vi "Set_Power_Unit.vi"(0 ".NET Reference in":refnum<k24>, 1 "unit":i32(ring) items=["dBm", "mW"], 3 "error in (no error)":errorcluster) -> (7 "Reference out":refnum<k24>, 10 "error out":errorcluster)   [LabVIEW 2017]
uses:
  LV_IL_Sample/DLL/InstrumentDLL.dll
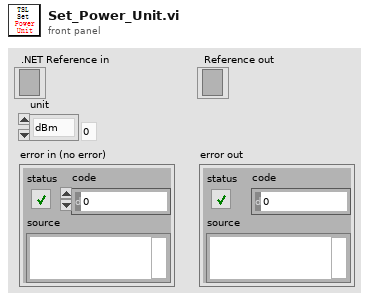
[diagram p1: front panel]
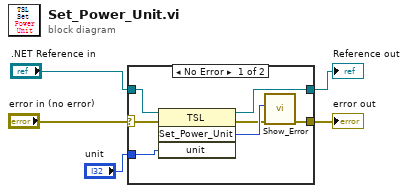
[diagram p0: block diagram]
diagram:
  n1 = case shown="No Error" "error in (no error)" {
    selector: "error in (no error)" -> [w6 w14]
    tunnel: ".NET Reference in" -> [w12 w13]
    tunnel: "unit" -> [w11 _]
    tunnel: [w10 w13] -> w4
    tunnel: [w7 w14] -> w3
    frame No Error {
      n2 = invoke on="调用节点" class="TSL" method="Set_Power_Unit"(reference=w12, error in=w6, "unit"=w11) -> (reference out=w10:refnum<k24>, error out=w8:errorcluster, "Set_Power_Unit"=w9:i32)  [unwired: 1 in, 1 out]
      n3 = call "Show_Error.vi"("error in (no error)"=w8, "Error"=w9) -> ("error out"=w7:errorcluster)  [unwired: 9 in]
    }
    frame Error {
    }
  }
  "Reference out" <- w4
  "error out" <- w3
